vi "MOCK_FP_Read_Double_Array.vi"(7 "Type":dbl[](array[numeric]), 8 "error in":errorcluster, 11 "FieldPoint IO Point In":refnum<k21>) -> (0 "error out":errorcluster, 1 "timestamp":dbl format="%.2f", 2 "Array":dbl[](array[numeric]) format="%#_13g", 3 "FieldPoint IO Point Out":refnum<k21>)   [LabVIEW 2017]
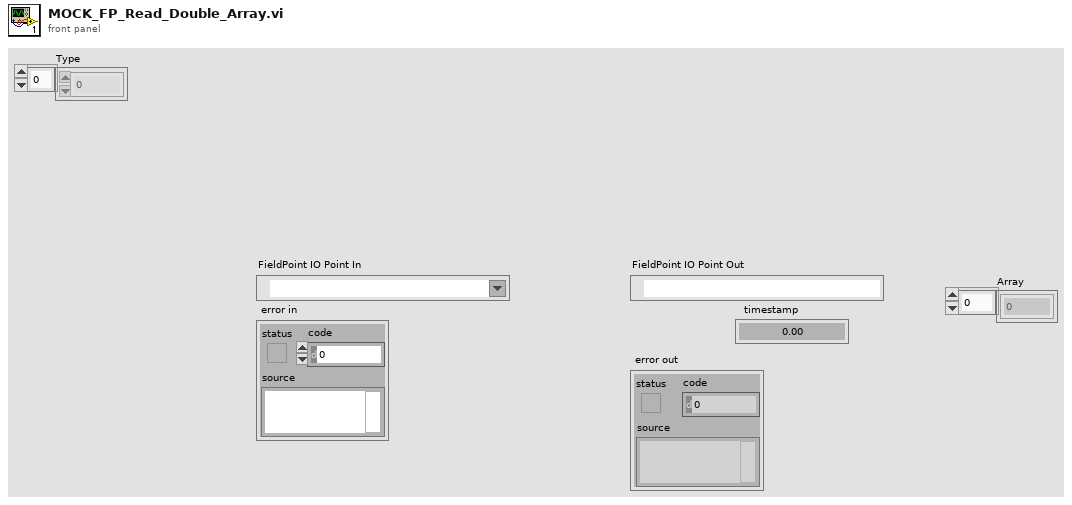
[diagram p1: front panel]
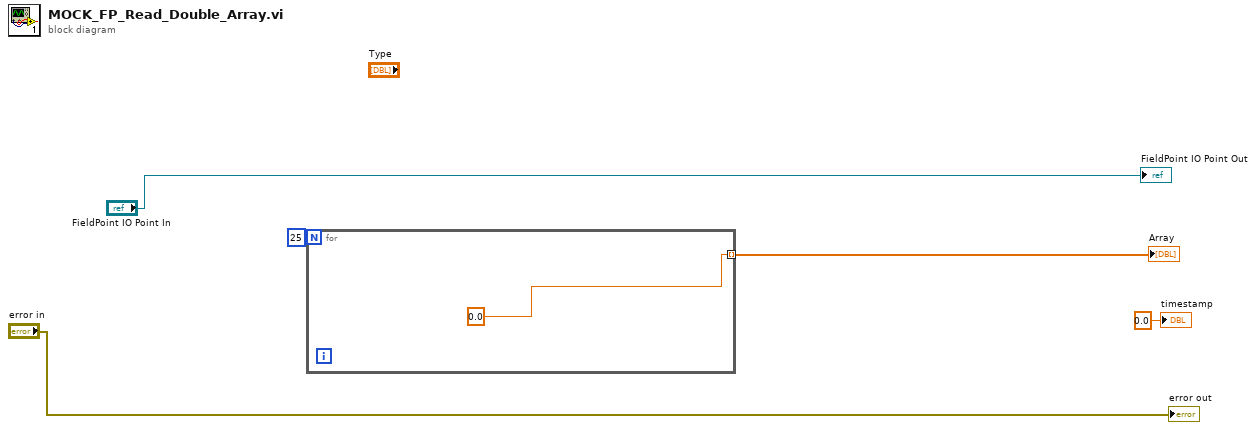
[diagram p0: block diagram]
diagram:
  n1 = for {
    N: 25 -> [_]
    tunnel: [0.0 ("f")] -> w2 mode=indexing
  }
  "Array" <- w2
  "FieldPoint IO Point Out" <- "FieldPoint IO Point In"
  "timestamp" <- 0.0 ("timestamp")
  "error out" <- "error in"
